vi "Put - Boolean.vi"(6 "timestamp":timestamp, 7 "PV name":string, 8 "error in (no error)":errorcluster, 9 "timeout":dbl[unit]=1.0, 10 "value":bool, 11 "Client in":refnum<class "Client.lvclass">) -> (0 "error out":errorcluster, 1 "timed out?":bool, 3 "Client out":refnum<class "Client.lvclass">)   [LabVIEW 2020, in "PV Access.lvlib" / "PVA Client.lvlib" / "Client.lvclass"]
uses:
  Client.lvclass
  Client.lvclass/Client.ctl
  09055bfe-3840-473e-8f73-dd572ee5ee6f.vi
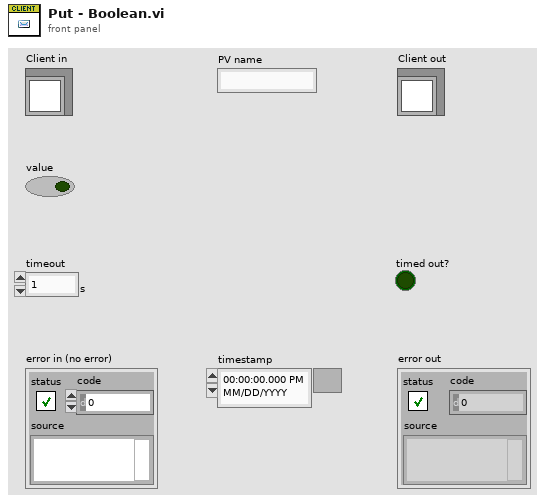
[diagram p1: front panel]
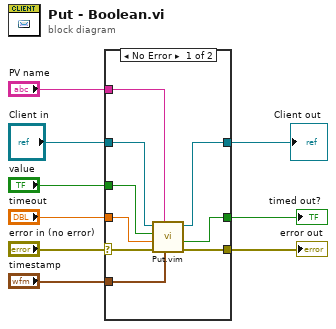
[diagram p0: block diagram]
diagram:
  n1 = case shown="No Error" "error in (no error)" {
    selector: "error in (no error)" -> [w12 w20]
    tunnel: [w11 w20] -> w8
    tunnel: [w13 w19] -> w6
    tunnel: "Client in" -> [w14 w19]
    tunnel: "value" -> [w18 _]
    tunnel: "timeout" -> [w17 _]
    tunnel: [w16 _] -> w3
    tunnel: "PV name" -> [w15 _]
    tunnel: "timestamp" -> [w10 _]
    frame No Error {
      n2 = call "Put.vim"("timestamp"=w10, "PV name"=w15, "error in"=w12, "timeout"=w17, "value"=w18, "Client in"=w14) -> ("error out"=w11:errorcluster, "timed out?"=w16:bool, "Client out"=w13:refnum<class "Client.lvclass">)  [unwired: 3 in]
    }
    frame Error {
    }
  }
  "error out" <- w8
  "Client out" <- w6
  "timed out?" <- w3
